vi "Create Report Info Tags.vi"(11 "Sequencer Module configuration in":refnum<class "Sequencer Module configuration.lvclass">) -> (3 "Array":refnum<class "TBM channel.lvclass">[](array[class]))   [LabVIEW 2015, in "Sequencer Module configuration.lvclass"]
uses:
  Sequencer Module configuration.lvclass
  <vilib>/NI/Tag Bus Module Framework/channel/TBM channel.lvclass
  <vilib>/NI/Tag Bus/tag/Data Type.ctl
  <vilib>/NI/Tag Bus Module Framework/channel/channel classification.ctl
  <vilib>/NI/Configuration Framework/serializable configuration/get alias.vi
  <vilib>/NI/Tag Bus/tag/tag descriptor.lvclass
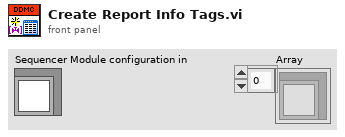
[diagram p1: front panel]
types:
  T1 = typedef "tag bus.lvlib/tag descriptor.lvclass/Data Type.ctl" = enum16{"Double", "Single", "I64", "I32", "I16", "I8", "U64", "U32", "U16", "U8", "Boolean", "String", "Array of Double", "Array of Single", "Array of I64", "Array of I32", "Array of I16", "Array of I8", "Array of U64", "Array of U32", "Array of U16", "Array of U8", "Array of Boolean", "Array of String"}
  T2 = typedef "TBM channel.lvclass/channel classification.ctl" = enum16{"input data", "output data", "processing parameter", "processing result"}
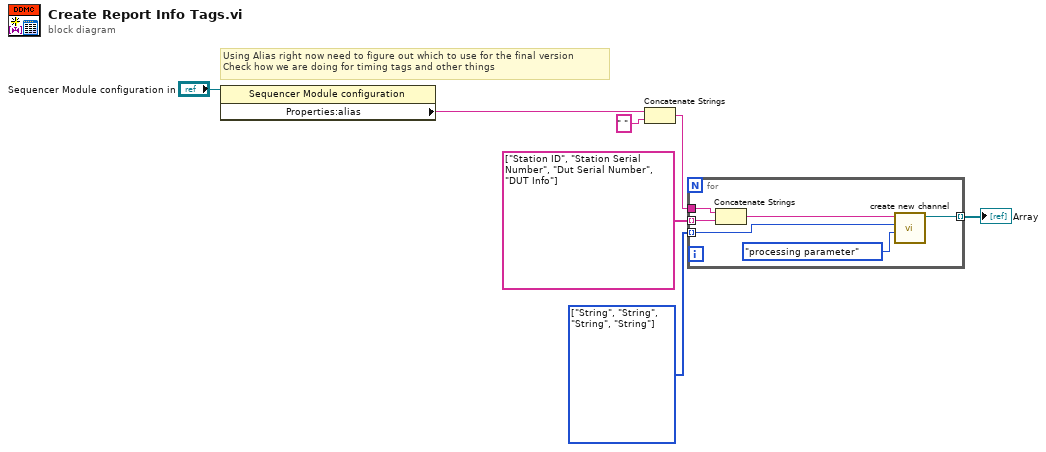
[diagram p0: block diagram]
diagram:
  w5 = T1[] [enum."String", enum."String", enum."String", enum."String"] items=["Double", "Single", "I64", "I32", "I16", "I8", "U64", "U32", "U16", "U8", "Boolean", "String", "Array of Double", "Array of Single", "Array of I64", "Array of I32", "Array of I16", "Array of I8", "Array of U64", "Array of U32", "Array of U16", "Array of U8", "Array of Boolean", "Array of String"]
  # "Using Alias right now need to figure out which to use for the final version\nCheck how we are doing for timing tags and other things"
  n1 = property class="Sequencer Module configuration"(reference="Sequencer Module configuration in") -> ("Properties:alias"=w3:string)  [unwired: 1 in, 2 out]
  n2 = Concatenate Strings(w3, " " ("string")) -> (w2:string)
  n3 = for {
    tunnel: [w8] -> w7 mode=indexing
    tunnel: w5 -> [w12] mode=indexing
    tunnel: string[] ["Station ID", "Station Serial Number", "Dut Serial Number", "DUT Info"] -> [w9] mode=indexing
    tunnel: w2 -> [w10]
    n4 = Concatenate Strings(w10, w9) -> (w11:string)
    n5 = call <vilib>:"create new channel.vi"("channel classification"=channel_classification."processing parameter", "data type"=w12, "channel name"=w11) -> ("channel"=w8:refnum<class "TBM channel.lvclass">)  [unwired: 8 in]
  }
  "Array" <- w7
